vi "BB_Siren_setup.vi"(8 "error in":errorcluster) -> (0 "error out":errorcluster, 2 "Sampling Info":cluster{"Fs":dbl, "#s":dbl}, 3 "task ID":T1 format="%.0x")   [LabVIEW 2015]
uses:
  <vilib>/sound2/lvsound2.llb/Sound Output Task ID.ctl
  <vilib>/sound2/lvsound2.llb/Sampling Mode.ctl
  <vilib>/sound2/lvsound2.llb/Sound Data Format.ctl
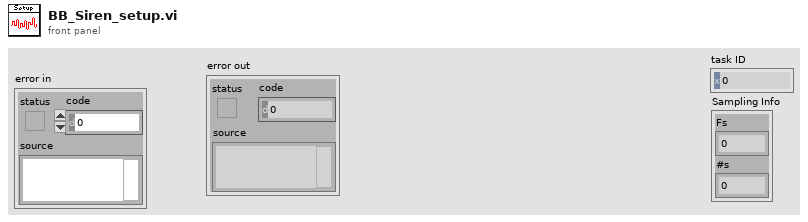
[diagram p1: front panel]
types:
  T1 = typedef "Sound Output Task ID.ctl" = u32
  T2 = typedef "Sound Data Format.ctl" = cluster{"sample rate (S/s)":dbl, "number of channels":i32, "bits per sample":i32}
  T3 = typedef "Sampling Mode.ctl" = i32
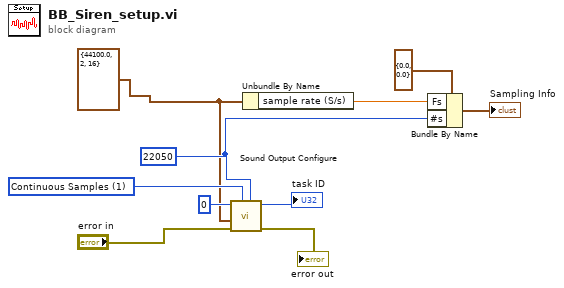
[diagram p0: block diagram]
diagram:
  w5 = T2 {"sample rate (S/s)"=44100.0, "number of channels"=2, "bits per sample"=16} ("Sound Format")
  w7 = 22050 ("Number of Samples/ch")
  w6 = T3 1 items=["Finite Samples", "Continuous Samples"] ("sample mode")
  n1 = call <vilib>:"Sound Output Configure.vi"("number of samples/ch"=w7, "sample mode"=w6, "error in (no error)"="error in", "sound format"=w5, "device ID"=u32 0 ("Device ID")) -> ("error out"=→"error out":errorcluster, "task ID"=→"task ID":T1)  [unwired: 5 in]
  n2 = Unbundle By Name(w5) -> ("sample rate (S/s)"=w8:dbl)
  n3 = Bundle By Name(cluster=cluster{"Fs":dbl, "#s":dbl} {"Fs"=0.0, "#s"=0.0} ("sampling info"), "Fs"=w8, "#s"=w7) -> (→"Sampling Info":cluster{"Fs":dbl, "#s":dbl})
